vi "Import from ProjFile Menu Entry.vi"(8 "error in (no error)":errorcluster, 9 "LangFile ref":refnum<data-value>, 10 "Menu Data":T1, 11 "LVProject File Path":path) -> (0 "error out":errorcluster, 3 "Menu Data out":refnum<class "Menu Data.lvclass">)   [LabVIEW 2013, in "SET Project Data.lvlib" / "Menu Data.lvclass"]
uses:
  Menu Data.lvclass
  Resource Data Class/Resource Data.lvclass
  Types/ProjFile_Menu Data.ctl
  Menu Data.lvclass/Menu Data.ctl
  SET Project Data.lvlib
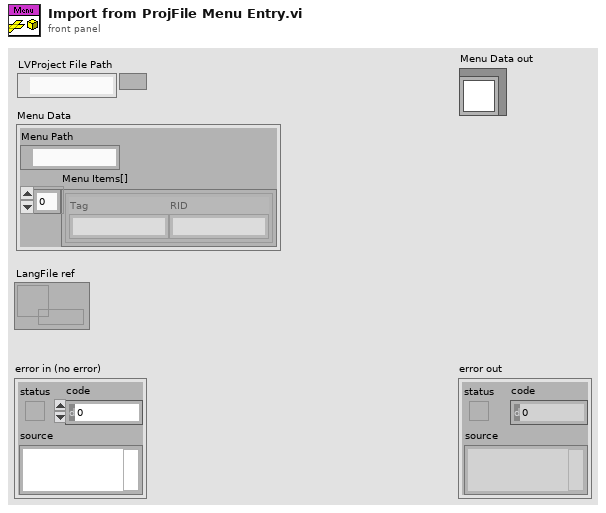
[diagram p1: front panel]
types:
  T1 = typedef "SET Project Data.lvlib/ProjFile_Menu Data.ctl" = cluster{"Menu Path":path, "Menu Items[]":cluster{"Tag":string, "RID":string}[]}
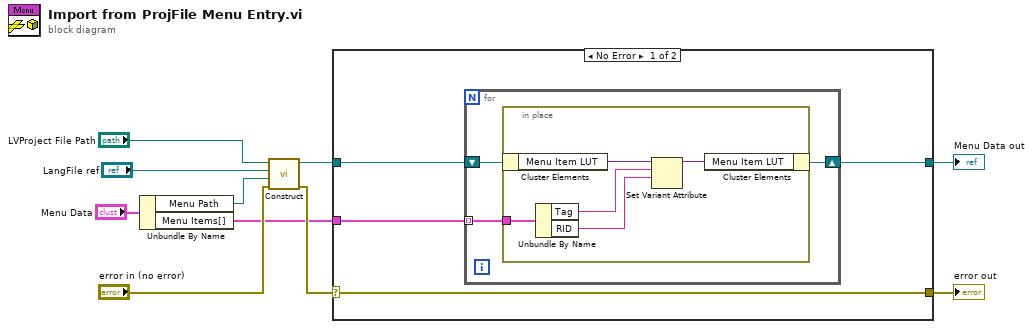
[diagram p0: block diagram]
diagram:
  n1 = Unbundle By Name("Menu Data") -> ("Menu Path"=w7:path, "Menu Items[]"=w2:cluster{"Tag":string, "RID":string}[])
  n2 = call "Construct.vi"("error in (no error)"="error in (no error)", "Menu Path (Relative)"=w7, "Resource Data ref"="LangFile ref", "LVProject File Path"="LVProject File Path") -> ("error out"=w5:errorcluster, "Menu Data out"=w3:refnum<class "Menu Data.lvclass">)  [unwired: 6 in]
  n3 = case shown="No Error" w5 {
    selector: w5 -> [w14 w24]
    tunnel: [w14 w24] -> w10
    tunnel: [w12 w23] -> w9
    tunnel: w3 -> [w13 w23]
    tunnel: w2 -> [w11 _]
    frame No Error {
      n4 = for {
        tunnel: w11 -> [w16] mode=indexing
        shift-right: [w15] -> w12
        shift-left: w13 -> [w17]
        n5 = in-place {
          in-place-border: w16 -> [w22]
          n6 = in-place-cluster #1(w17) -> ("Menu Item LUT"=w21:variant)
          n7 = Unbundle By Name(w22) -> ("Tag"=w19:string, "RID"=w18:string)
          n8 = Set Variant Attribute(Variant=w21, name=w19, value=w18) -> (Variant out=w20:variant)  [unwired: 1 in, 2 out]
          n9 = in-place-cluster #1("Menu Item LUT"=w20) -> (w15:refnum<class "Menu Data.lvclass">)
        }
      }
    }
    frame Error {
    }
  }
  "error out" <- w10
  "Menu Data out" <- w9
